vi "GT Get Thread Sts.vi"(8 "error in (no error)":errorcluster caption="错误输入（无错误）", 9 "pThreadSts":T1, 10 "thread":i16, 11 "cardNum":i16) -> (0 "error out":errorcluster caption="错误输出", 1 "pThreadSts out":T1, 3 "function return":i16)   [LabVIEW 2020, in "gts.lvlib"]
doc: "GT_API GT_GetThreadSts(short cardNum,short thread,TThreadSts *pThreadSts);"
uses:
  gts.lvlib
  dll/32bit/multi_card/gts.dll
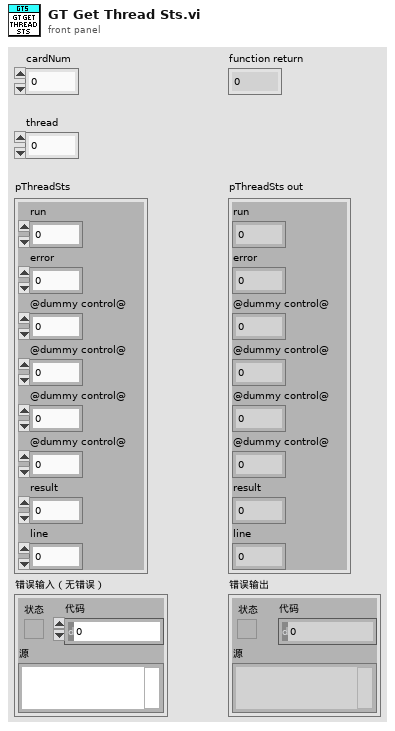
[diagram p1: front panel]
types:
  T1 = cluster{"run":i16, "error":i16, "@dummy control@":i8, "@dummy control@":i8, "@dummy control@":i8, "@dummy control@":i8, "result":dbl, "line":i16}
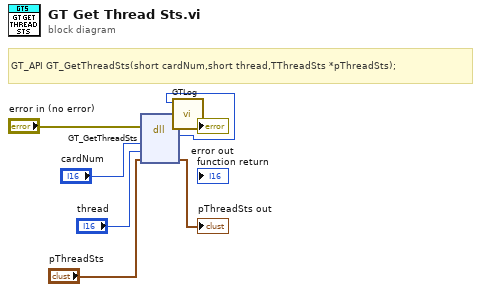
[diagram p0: block diagram]
diagram:
  # "GT_API GT_GetThreadSts(short cardNum,short thread,TThreadSts *pThreadSts);"
  n1 = dll-call lib="C:/1228/dll/32bit/multi_card/gts.dll" fn="GT_GetThreadSts"(error in="error in (no error)", "cardNum"="cardNum", "thread"="thread", "pThreadSts"="pThreadSts") -> (error out=w3:errorcluster, w1:i16, "pThreadSts"=→"pThreadSts out":T1)  [unwired: 4 in, 1 out]
  n2 = call "GTLog.vi"("error in (no error)"=w3, "Numeric"=w1) -> ("error out"=→"error out":errorcluster)  [unwired: 9 in]
